vi "old_XML_Get_General_Settings.vi"(8 "error in (no error)":errorcluster, 11 "reference out":refnum<k24>) -> (0 "error out":errorcluster, 2 "General Settings":T1={"Communication_Type"=0, "Modbus_Type"=0, "Read_Write_Loop_Period"=-1, "TCP Settings"={"TCP_Settings_Port"=0, "TCP_Settings_IP_Timeout"=0, "TCP_Settings_IP_Slave_Address"=""}, "Serial Settings"={"Serial_Settings_Flow_Control"=0, "Serial_Settings_Baud_Rate"=0, "Serial_Settings_Parity"=0, "Serial_Settings_Resource_Name"="", "Serial_Settings_Serial_Type"=0, "Serial_Settings_Unit_ID"=0}} {"Communication_Type" items=["TCP", "Serial"]; "Modbus_Type" items=["Master", "Slave"]; "Serial Settings"."Serial_Settings_Flow_Control" items=["None", "XONXOFF", "RTSCTS", "XONXOFFANDRTSCTS", "DTRDSR", "XONXOFFANDDTRDSR"]; "Serial Settings"."Serial_Settings_Parity" items=["None", "Odd", "Even"]; "Serial Settings"."Serial_Settings_Serial_Type" items=["RTU", "ASCII"]}, 3 "reference out":refnum<k24>)   [LabVIEW 2013, in "Modbus System Explorer.lvlib" / "XML_Deserializer.lvlib"]
uses:
  XML_Deserializer.lvlib
  Controls/Modbus_General_Settings.ctl
  Controls/Modbus_Communication_Type.ctl
  Controls/Modbus_Type.ctl
  Controls/Modbus_Serial_Settings_Flow_Control.ctl
  Controls/Modbus_Serial_Settings_Parity.ctl
  Controls/Modbus_Serial_Settings_Serial_Type.ctl
  D:/NI/Sales/Canada/Sales/2014/Mon Espace/Modbus Custom-Device/XML Deserializer/XML VIs/API/Sub-VIs/Modbus_CD_XML.dll
  Modbus_CD_XML.dll
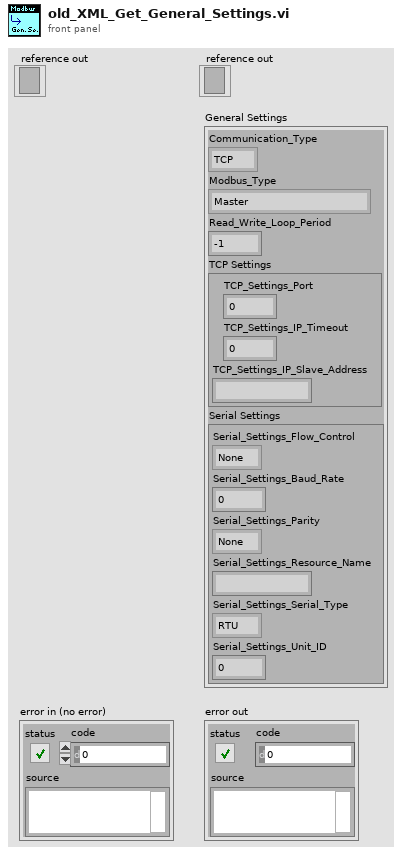
[diagram p1: front panel]
types:
  T1 = typedef "Modbus System Explorer.lvlib/XML_Deserializer.lvlib/Modbus_General_Settings.ctl" = cluster{"Communication_Type":T2, "Modbus_Type":T3, "Read_Write_Loop_Period":i64, "TCP Settings":cluster{"TCP_Settings_Port":u16, "TCP_Settings_IP_Timeout":u32, "TCP_Settings_IP_Slave_Address":string}, "Serial Settings":cluster{"Serial_Settings_Flow_Control":T4, "Serial_Settings_Baud_Rate":u32, "Serial_Settings_Parity":T5, "Serial_Settings_Resource_Name":string, "Serial_Settings_Serial_Type":T6, "Serial_Settings_Unit_ID":i8}}
  T2 = typedef "Modbus System Explorer.lvlib/XML_Deserializer.lvlib/Modbus_Communication_Type.ctl" = i32
  T3 = typedef "Modbus System Explorer.lvlib/XML_Deserializer.lvlib/Modbus_Type.ctl" = i32
  T4 = typedef "Modbus System Explorer.lvlib/XML_Deserializer.lvlib/Modbus_Serial_Settings_Flow_Control.ctl" = i32
  T5 = typedef "Modbus System Explorer.lvlib/XML_Deserializer.lvlib/Modbus_Serial_Settings_Parity.ctl" = i32
  T6 = typedef "Modbus System Explorer.lvlib/XML_Deserializer.lvlib/Modbus_Serial_Settings_Serial_Type.ctl" = i32
  T7 = cluster{"Communication_Type":i32, "Modbus_Type":i32, "Read_Write_Loop_Period":i64, "TCP Settings":cluster{"TCP_Settings_Port":u16, "TCP_Settings_IP_Timeout":u32, "TCP_Settings_IP_Slave_Address":string}, "Serial Settings":cluster{"Serial_Settings_Flow_Control":i32, "Serial_Settings_Baud_Rate":u32, "Serial_Settings_Parity":i32, "Serial_Settings_Resource_Name":string, "Serial_Settings_Serial_Type":i32, "Serial_Settings_Unit_ID":i8}}
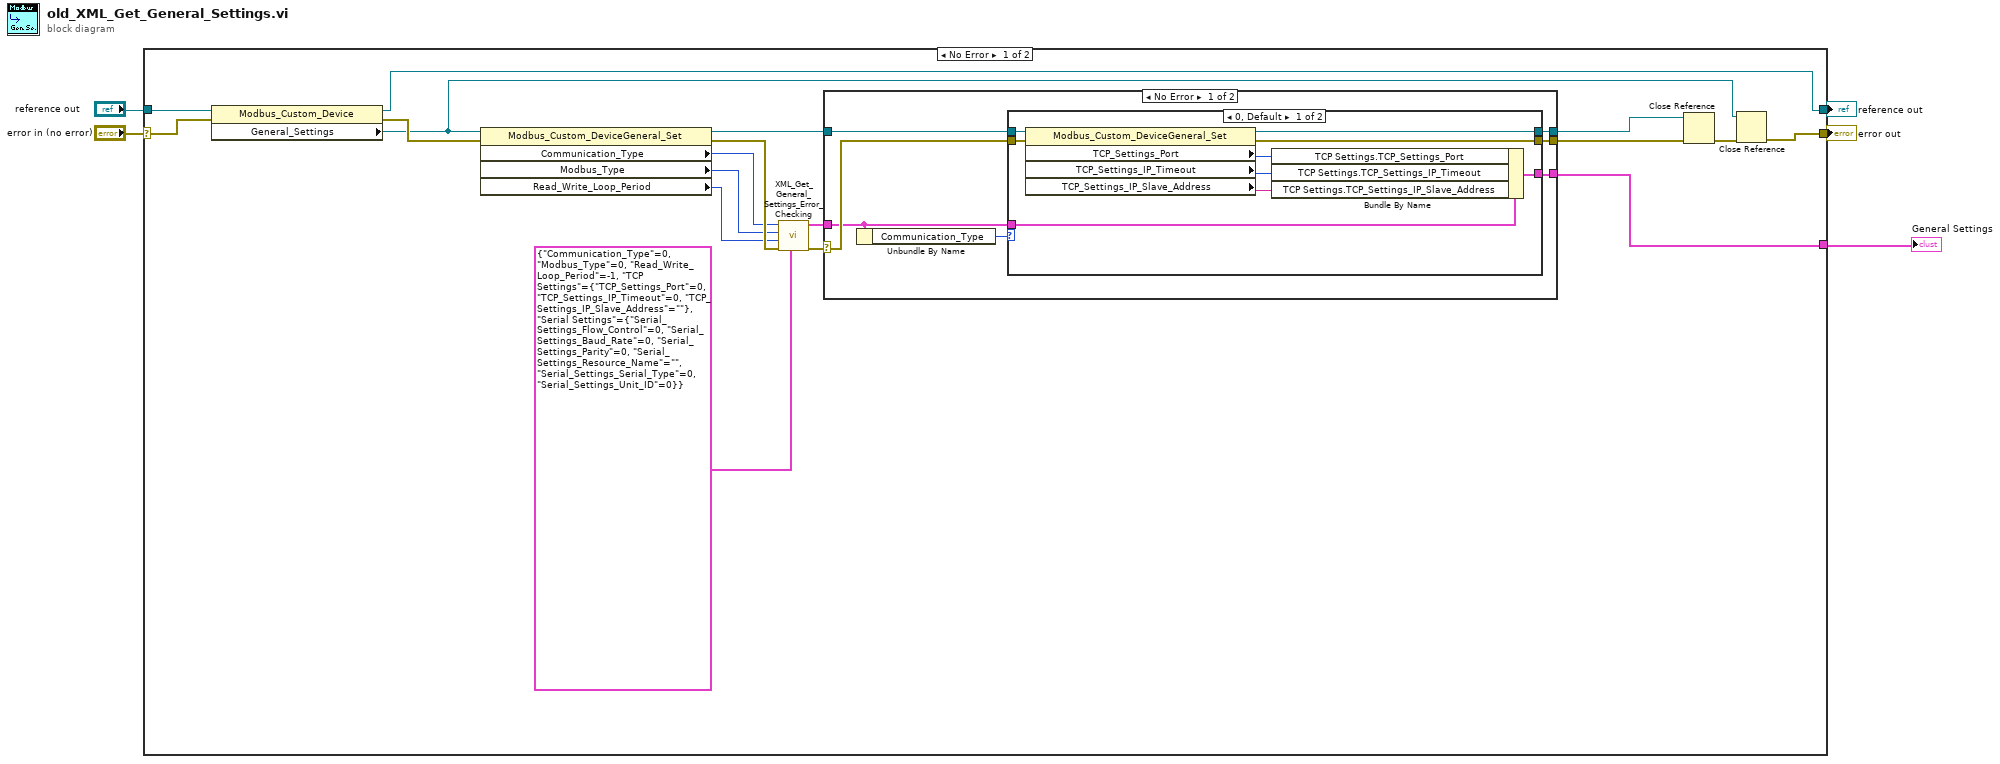
[diagram p0: block diagram]
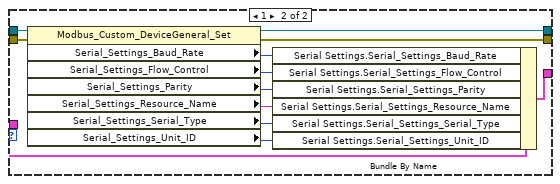
[diagram p2: hidden frame]
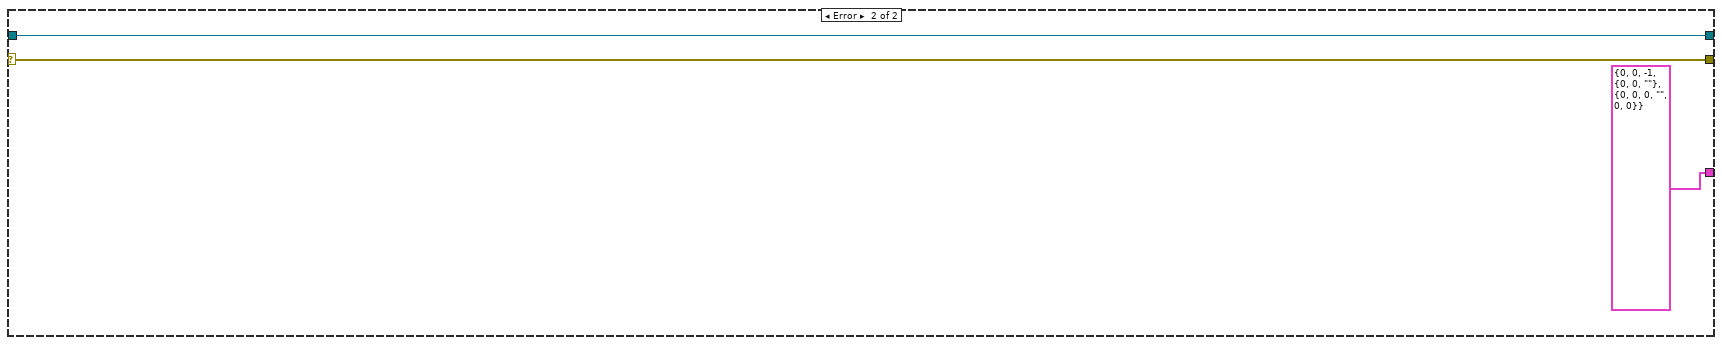
[diagram p4: hidden frame]
diagram:
  n1 = case shown="No Error" "error in (no error)" {
    selector: "error in (no error)" -> [w17 w56]
    tunnel: "reference out" -> [w20 w57]
    tunnel: [w19 w56] -> w2
    tunnel: [w18 w57] -> w3
    tunnel: [w13 T7 {"Communication_Type"=0, "Modbus_Type"=0, "Read_Write_Loop_Period"=-1, "TCP Settings"={"TCP_Settings_Port"=0, "TCP_Settings_IP_Timeout"=0, "TCP_Settings_IP_Slave_Address"=""}, "Serial Settings"={"Serial_Settings_Flow_Control"=0, "Serial_Settings_Baud_Rate"=0, "Serial_Settings_Parity"=0, "Serial_Settings_Resource_Name"="", "Serial_Settings_Serial_Type"=0, "Serial_Settings_Unit_ID"=0}} ("General Settings")] -> w5
    frame No Error {
      n2 = property class="Modbus_Custom_Device"(reference=w20, error in=w17) -> (reference out=w18:refnum<k24>, error out=w23:errorcluster, "General_Settings"=w21:refnum<k24>)
      n3 = property class="Modbus_Custom_DeviceGeneral_Set"(reference=w21, error in=w23) -> (reference out=w16:refnum<k24>, error out=w12:errorcluster, "Communication_Type"=w9:i32, "Modbus_Type"=w8:i32, "Read_Write_Loop_Period"=w7:i64)
      n4 = call "XML_Get_General_Settings_Error_Checking.vi"("General Settings"=T1 {"Communication_Type"=0, "Modbus_Type"=0, "Read_Write_Loop_Period"=-1, "TCP Settings"={"TCP_Settings_Port"=0, "TCP_Settings_IP_Timeout"=0, "TCP_Settings_IP_Slave_Address"=""}, "Serial Settings"={"Serial_Settings_Flow_Control"=0, "Serial_Settings_Baud_Rate"=0, "Serial_Settings_Parity"=0, "Serial_Settings_Resource_Name"="", "Serial_Settings_Serial_Type"=0, "Serial_Settings_Unit_ID"=0}}, "error in (no error)"=w12, "Read_Write_Loop_Period"=w7, "Modbus_Type"=w8, "Communication_Type"=w9) -> ("error out"=w6:errorcluster, "General Settings"=w11:T1)  [unwired: 5 in]
      n5 = case shown="No Error" w6 {
        selector: w6 -> [w26 w52]
        tunnel: w16 -> [w30 w53]
        tunnel: [w29 w52] -> w15
        tunnel: [w28 w53] -> w14
        tunnel: [w27 w54] -> w13
        tunnel: w11 -> [w25 w54]
        frame No Error {
          n6 = Unbundle By Name(w25) -> ("Communication_Type"=w24:T2)
          n7 = case shown="0, Default" w24 {
            tunnel: w30 -> [w31 w51]
            tunnel: w26 -> [w39 w50]
            tunnel: [w38 w49] -> w29
            tunnel: [w37 w48] -> w28
            tunnel: w25 -> [w36 w47]
            tunnel: [w32 w40] -> w27
            frame 0, Default {
              n8 = property class="Modbus_Custom_DeviceGeneral_Set"(reference=w31, error in=w39) -> (reference out=w37:refnum<k24>, error out=w38:errorcluster, "TCP_Settings_Port"=w35:u16, "TCP_Settings_IP_Timeout"=w34:u32, "TCP_Settings_IP_Slave_Address"=w33:string)
              n9 = Bundle By Name(cluster=w36, "TCP Settings.TCP_Settings_Port"=w35, "TCP Settings.TCP_Settings_IP_Timeout"=w34, "TCP Settings.TCP_Settings_IP_Slave_Address"=w33) -> (w32:T1)
            }
            frame 1 {
              n10 = property class="Modbus_Custom_DeviceGeneral_Set"(reference=w51, error in=w50) -> (reference out=w48:refnum<k24>, error out=w49:errorcluster, "Serial_Settings_Baud_Rate"=w46:u32, "Serial_Settings_Flow_Control"=w45:i32, "Serial_Settings_Parity"=w44:i32, "Serial_Settings_Resource_Name"=w43:string, "Serial_Settings_Serial_Type"=w42:i32, "Serial_Settings_Unit_ID"=w41:i8)
              n11 = Bundle By Name(cluster=w47, "Serial Settings.Serial_Settings_Baud_Rate"=w46, "Serial Settings.Serial_Settings_Flow_Control"=w45, "Serial Settings.Serial_Settings_Parity"=w44, "Serial Settings.Serial_Settings_Resource_Name"=w43, "Serial Settings.Serial_Settings_Serial_Type"=w42, "Serial Settings.Serial_Settings_Unit_ID"=w41) -> (w40:T1)
            }
          }
        }
        frame Error {
        }
      }
      n12 = Close Reference(reference=w14, error in (no error)=w15) -> (error out=w22:errorcluster)
      n13 = Close Reference(reference=w21, error in (no error)=w22) -> (error out=w19:errorcluster)
    }
    frame Error {
    }
  }
  "General Settings" <- w5
  "reference out" <- w3
  "error out" <- w2
